vi "Add Sample.vi"(6 "Labels":map{string, string}(c390), 8 "error in (no error)":errorcluster, 9 "Timestamp":timestamp format="%<%x %.3X>T", 10 "Value":dbl, 11 "Metric in":refnum<class "Metric.lvclass">) -> (0 "error out":errorcluster, 3 "Metric out":refnum<class "Metric.lvclass">)   [LabVIEW 2020, in "Metrics.lvlib" / "Metric.lvclass"]
uses:
  Metric.lvclass
  <vilib>/Utility/miscctls.llb/LVMapReplaceAction.ctl
  Metric.lvclass/Metric.ctl
  sample/Sample.lvclass
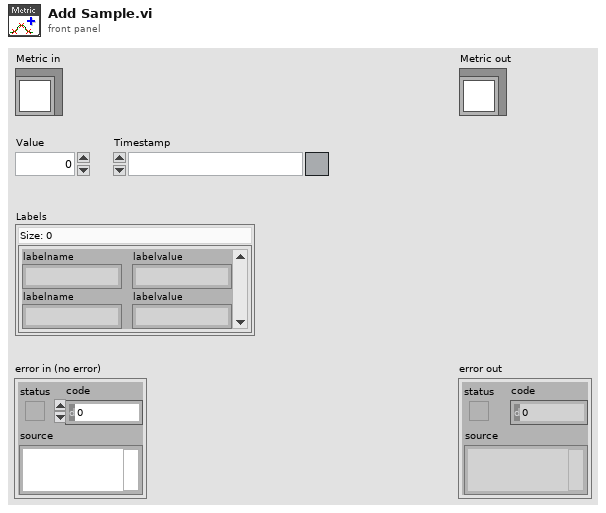
[diagram p1: front panel]
types:
  T1 = typedef "LVMapReplaceAction.ctl" = enum32{"Modify Entry only if found", "Add or Modify Entry", "Delete Entry"}
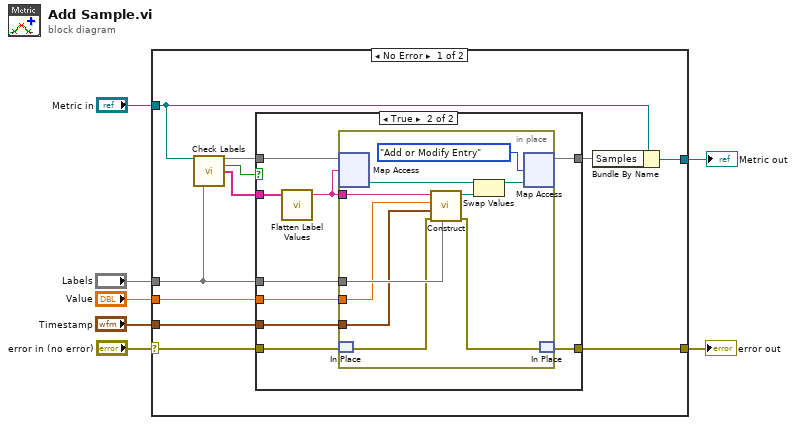
[diagram p0: block diagram]
diagram:
  n1 = case shown="No Error" "error in (no error)" {
    selector: "error in (no error)" -> [w10 w41]
    tunnel: [w11 w41] -> w6
    tunnel: [w12 w40] -> w4
    tunnel: "Metric in" -> [w14 w40]
    tunnel: "Value" -> [w16 _]
    tunnel: "Timestamp" -> [w15 _]
    tunnel: "Labels" -> [w8 _]
    frame No Error {
      n2 = call-dynamic "Check Labels.vi"("Metric in"=w14, "Labels"=w8) -> ("Samples"=w17:map{string, refnum<class "Sample.lvclass">}, "Valid Labels"=w18:bool, "Label Values"=w9:string[])  [unwired: 10 in, 1 out]
      n3 = case shown="True" w18 {
        tunnel: w17 -> [w19 w22]
        tunnel: [w19 w28] -> w13
        tunnel: w16 -> [_ w27]
        tunnel: w15 -> [_ w26]
        tunnel: w8 -> [_ w25]
        tunnel: [w20 w24] -> w11
        tunnel: w10 -> [w20 w23]
        tunnel: w9 -> [_ w21]
        frame False {
        }
        frame True {
          n4 = call "Flatten Label Values.vi"("Label Values"=w21) -> ("Flattened labelvalues"=w29:string)  [unwired: 4 in]
          n5 = in-place {
            in-place-border: w29 -> [w37]
            in-place-border: w27 -> [w36]
            in-place-border: w26 -> [w35]
            in-place-border: w25 -> [w39]
            n6 = in-place-map #1(w22, w29) -> (w31:refnum<class "Sample.lvclass">)  [unwired: 1 in, 1 out]
            n7 = in-place-match #2(w23) -> (w33:errorcluster)
            n8 = call "Construct.vi"("Labels"=w39, "error in (no error)"=w33, "Timestamp"=w35, "Value"=w36, "Name"=w37) -> ("error out"=w34:errorcluster, "Sample out"=w32:refnum<class "Sample.lvclass">)  [unwired: 5 in]
            n9 = Swap Values(12:w31, 14:w32) -> (1:w30:refnum<class "Sample.lvclass">)  [unwired: 1 in, 1 out]
            n10 = in-place-map #1(w30, LVMapReplaceAction."Add or Modify Entry" ("action")) -> (w28:map{string, refnum<class "Sample.lvclass">})  [unwired: 2 out]
            n11 = in-place-match #2(w34) -> (w24:errorcluster)
          }
        }
      }
      n12 = Bundle By Name(cluster=w14, "Samples"=w13) -> (w12:refnum<class "Metric.lvclass">)
    }
    frame Error {
    }
  }
  "error out" <- w6
  "Metric out" <- w4
